vi "PWM Counter.vi"(0 "PWM Output Pin":refnum<k21>="PWM Value 1", 1 "PWM Enable":refnum<k21>="PWM Enable 1", 2 "PWM Value":refnum<k21>="PWM Value 1") -> ()   [LabVIEW 2024]
uses:
  <vilib>/rvi/DataTransferAndStorage/Container/XNode/niFpgaContainer.xnode
  <vilib>/rvi/DataTransferAndStorage/Register/Emulation/niFpgaRegisterEmulationRefIn.vi
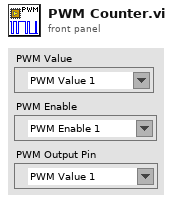
[diagram p1: front panel]
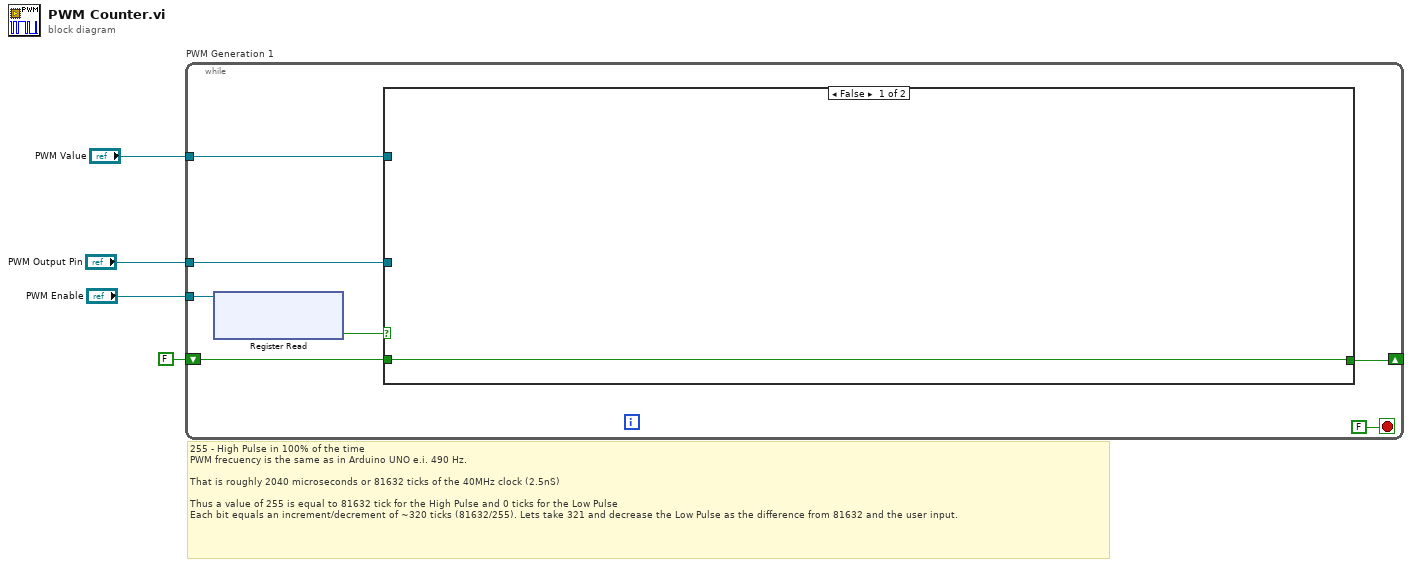
[diagram p0: block diagram]
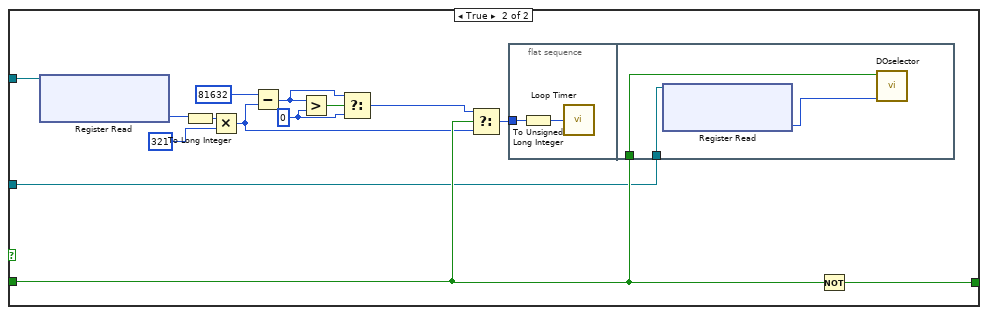
[diagram p2: hidden frame]
diagram:
  # "255 - High Pulse in 100% of the time\nPWM frecuency is the same as in Arduino UNO e.i. 490 Hz.\n\nThat is roughly 2040 microseconds or 81632 ticks of the 40MHz clock (2.5nS)\n\nThus a value of 255 is equal to 81632 tick for the High Pulse and 0 ticks for the Low Pulse\nEach bit equals an increment/decrement of ~320 ticks (81632/255). Lets take 321 and decrease the Low Pulse as the difference from 81632 and the user input."
  n1 = while "PWM Generation 1" {
    shift-right: [w10] -> _
    shift-left: FALSE -> [w11]
    tunnel: "PWM Enable" -> [w9]
    tunnel: "PWM Value" -> [w8]
    tunnel: "PWM Output Pin" -> [w7]
    stop <- FALSE stop-if-true
    n2 = xnode ("Register Read")("Register In"=w9) -> ("Data"=w5:bool)  [unwired: 1 out]
    n3 = case shown="False" w5 {
      tunnel: w11 -> [w12 w25]
      tunnel: [w12 w24] -> w10
      tunnel: w8 -> [_ w15]
      tunnel: w7 -> [_ w13]
      frame False {
      }
      frame True {
        w16 = 0 ("y")
        n4 = xnode ("Register Read")("Register In"=w15) -> ("Data"=w14:u8)  [unwired: 1 out]
        n5 = To Long Integer(number=w14) -> (32bit integer=w22:i32)
        n6 = Multiply(x=w22, y=321) -> (x*y=w17:i32)
        n7 = Subtract(x=81632, y=w17) -> (x-y=w19:i32)
        n8 = Greater?(x=w19, y=w16) -> (0:w20:bool)
        n9 = Select(t=w19, s=w20, f=w16) -> (s? t:f=w18:i32)
        n10 = Select(t=w18, s=w25, f=w17) -> (s? t:f=w26:i32)
        n11 = flat-sequence {
          tunnel: w26 -> [w28]
          tunnel: w25 -> [w31]
          tunnel: w13 -> [w29]
          frame #0 {
            n12 = To Unsigned Long Integer(number=w28) -> (unsigned 32bit integer=w27:u32)
            n13 = call "Loop Timer"("Count(Ticks)"=w27) -> ()  [unwired: 1 out]
          }
          frame #1 {
            n14 = xnode ("Register Read")("Register In"=w29) -> ("Data"=w30:u8)  [unwired: 1 out]
            n15 = call "DOselector.vi"("I/O element"=w30, "value"=w31) -> ()  [unwired: 10 in]
          }
        }
        n16 = Not(x=w25) -> (.not. x?=w24:bool)
      }
    }
  }
